vi "Next Step.vi"(8 "error in (no error)":errorcluster, 11 "Varian Continuous in":refnum<class "Varian Continuous.lvclass">) -> (0 "error out":errorcluster, 1 "Current Step":u32, 2 "Current Position":dbl, 3 "Varian Continuous out":refnum<class "Varian Continuous.lvclass">)   [LabVIEW 2009, in "Varian Continuous.lvclass"]
doc: "(Dynamic) Move to the next preconfigured step of this Scanner, and return the current position (actual, not intended) of this Scanner. Increment the step counter by one."
uses:
  Varian Continuous.lvclass
  Scanner/Scanner.lvclass
  <vilib>/DAQmx/create/channels.llb/DAQmx Create Channel (AO-Voltage-Basic).vi
  Instruments/Varian Magnet/Varian Max Field.vi
  Instruments/Varian Magnet/Varian Magnet.lvclass
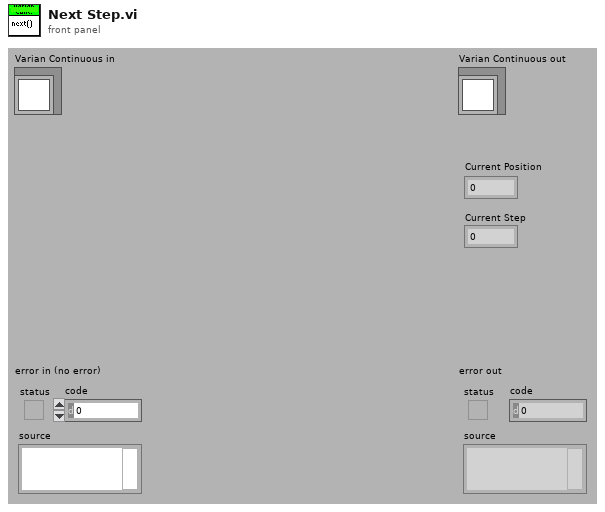
[diagram p1: front panel]
types:
  T1 = typedef "Scanner.lvclass/Range.ctl" = cluster{"xi":dbl, "xf":dbl, "dx":dbl, "Return to...?":bool, "Return to":dbl}
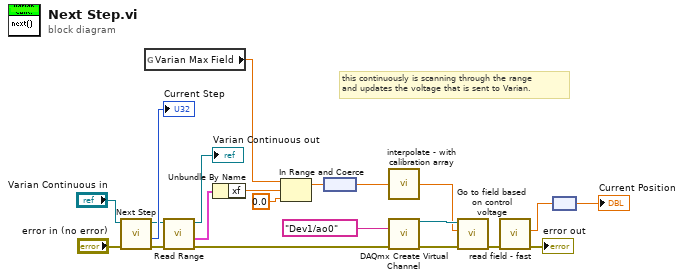
[diagram p0: block diagram]
diagram:
  # "this continuously is scanning through the range\nand updates the voltage that is sent to Varian."
  n1 = call-parent "Next Step.vi"("error in (no error)"="error in (no error)", "Scanner in"="Varian Continuous in") -> ("error out"=w4:errorcluster, "Current Step"=→"Current Step":u32, "Scanner out"=w6:refnum<class "Varian Continuous.lvclass">)  [unwired: 7 out]
  n2 = global read "Varian Max Field.vi" "Varian Max Field"() -> (w10:dbl[unit])
  n3 = call-dynamic "Read Range.vi"("error in (no error)"=w4, "Scanner.lvclass in"=w6) -> ("error out"=w3:errorcluster, "Range"=w2:T1, "Scanner.lvclass out"=→"Varian Continuous out":refnum<class "Varian Continuous.lvclass">)  [unwired: 4 in, 3 out]
  n4 = Unbundle By Name(w2) -> ("xf"=w1:dbl)
  n5 = In Range and Coerce(upper limit=w10, x=w1, lower limit=dbl[unit] 0.0) -> (coerced(x)=w8:dbl[unit])  [unwired: 1 out]
  n6 = node(w8) -> (w11:dbl)
  n7 = call "interpolate - with calibration array.vi"("Input Number"=w11) -> ("Interpolated Function Value"=w7:dbl)
  n8 = call-poly <vilib>:"DAQmx Create Virtual Channel.vi"("physical channels"=tag "Dev1/ao0", "error in"=w3) -> ("task out"=w12:refnum<k21>, "error out"=w14:errorcluster)  [unwired: 7 in, 5 out]
  n9 = call "Go to field based on control voltage.vi"("error in"=w14, "Control Voltage"=w7, "task in"=w12) -> ("error out"=w13:errorcluster)  [unwired: 7 in, 1 out]
  n10 = call "read field - fast.vi"("error in (no error)"=w13) -> ("error out"=→"error out":errorcluster, "Current field (T)"=w16:dbl[unit])  [unwired: 8 in, 1 out]
  n11 = node(w16) -> (→"Current Position":dbl)
